vi "Prepare Execution.vi"(0 "Session Handle in":T2, 11 "error in (no error)":errorcluster) -> (4 "Session Handle out":T2, 8 "Execution":T1, 15 "error out":errorcluster)   [LabVIEW 2019, in "HTS.lvlib" / "Engine.lvclass"]
uses:
  Engine.lvclass
  Execution/Execution.lvclass
  Typedefs/Session Handle.ctl
  Execution/Typedefs/Session Handle.ctl
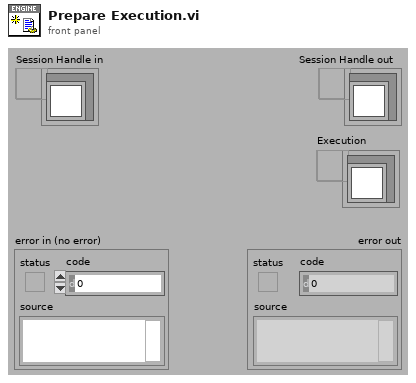
[diagram p1: front panel]
types:
  T1 = typedef "HTS.lvlib/Execution.lvclass/Session Handle.ctl" = refnum<data-value>
  T2 = typedef "HTS.lvlib/Engine.lvclass/Session Handle.ctl" = refnum<data-value>
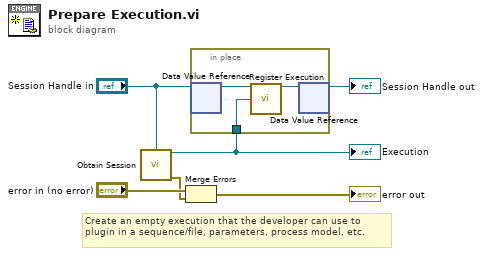
[diagram p0: block diagram]
diagram:
  # "Create an empty execution that the developer can use to plugin in a sequence/file, parameters, process model, etc."
  n1 = call "Obtain Session.vi"("Engine"="Session Handle in") -> ("Session Handle"=w4:T1, "error out"=w1:errorcluster)  [unwired: 13 in]
  "Execution" <- w4
  n2 = Merge Errors("error in (no error)", w1) -> (→"error out":errorcluster)
  n3 = in-place {
    in-place-border: w4 -> [w7]
    n4 = in-place-dvr #1("Session Handle in") -> (w9:refnum<class "Engine.lvclass">)  [unwired: 1 out]
    n5 = call "Register Execution.vi"("Engine in"=w9, "Execution"=w7) -> ("Engine out"=w8:refnum<class "Engine.lvclass">)  [unwired: 12 in, 1 out]
    n6 = in-place-dvr #1(w8) -> (→"Session Handle out":T2)  [unwired: 1 out]
  }
